vi "ConfigureScaler.vi"(8 "error in (no error)":errorcluster, 10 "handle":i32, 11 "VME Base Address":u32) -> (0 "error out":errorcluster, 2 "VME Base Address out":u32, 3 "handle out":i32)   [LabVIEW 2014]
uses:
  Program Files (x86)/CAEN/Comm/labview/CAENComm.lvlib
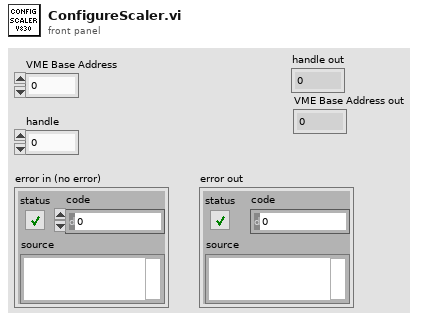
[diagram p1: front panel]
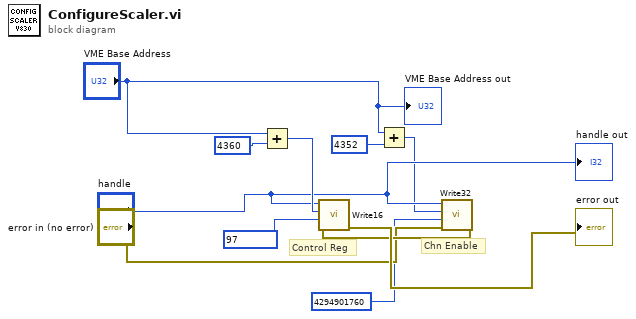
[diagram p0: block diagram]
diagram:
  # "Chn Enable"
  # "Control Reg"
  n1 = Add(x="VME Base Address", y=u32 4360) -> (x+y=w7:u32)
  n2 = Add(x="VME Base Address", y=u32 4352) -> (x+y=w3:u32)
  n3 = call "Write32.vi"("error in (no error)"="error in (no error)", "Data"=u32 4294901760, "Address"=w3, "handle"="handle") -> ("error out"=w10:errorcluster)  [unwired: 7 in]
  n4 = call "Write16.vi"("error in (no error)"=w10, "Data"=u16 97, "Address"=w7, "handle"="handle") -> ("error out"=→"error out":errorcluster)  [unwired: 7 in]
  "handle out" <- "handle"
  "VME Base Address out" <- "VME Base Address"
